vi "DHTxx Temp-Humidity Sensor.vi"   [LabVIEW 2014]
uses:
  QwaveSys_Interface/QwaveSys_Interface.lvlib
  QwaveSys_ESP8266/QwaveSys_ESP8266.lvlib
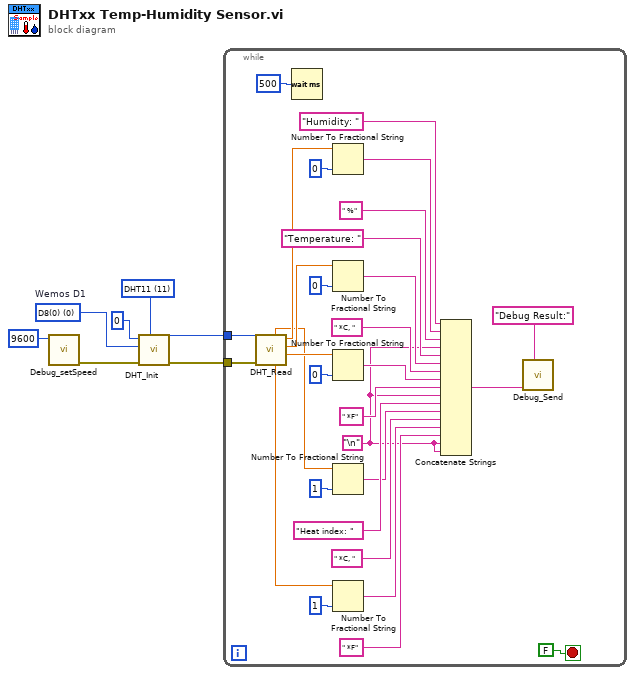
[diagram p0: block diagram]
diagram:
  w2 = u8 0 items=["D0-RX(3)"=3, "D1-TX(1)"=1, "D2(16)"=16, "D3/D15/SCL(5)"=5, "D4/D14/SDA(4)"=4, "D5/D13/SCK(14)-(LED)"=14, "D6/D12/MISO(12)"=12, "D7/D11/MOSI(13)"=13, "D8(0)"=0, "D9/TX1(2)"=2, "D10/SS (15)"=15, "ADC0,(17)"=17]  # Wemos D1
  w4 = u16 11 items=["DHT11"=11, "DHT21"=21, "DHT22"=22] ("Type")
  n1 = call "Debug_setSpeed.vi"("Speed"=u32 9600) -> ("error out"=w1:errorcluster)  [unwired: 10 in]
  n2 = call "DHT_Init.vi"("Type"=w4, "error in (no error)"=w1, "PIN"=w2, "Interface (0-4)"=u8 0) -> ("error out"=w6:errorcluster, "Instance"=w5:u8)  [unwired: 6 in]
  n3 = while {
    tunnel: w6 -> [w37]
    tunnel: w5 -> [w8]
    stop <- FALSE stop-if-true
    w11 = "\n" ("Line Feed Constant")
    n4 = call "DHT_Read.vi"("Instance"=w8, "error in (no error)"=w37) -> ("Fahrenheit"=w24:dbl, "Celsius"=w25:dbl, "Humidity"=w31:dbl, "Heat Index (Fahrenheit)"=w22:dbl, "Heat Index (Celsius)"=w23:dbl)  [unwired: 4 in, 1 out]
    n5 = Wait (ms)(milliseconds to wait=u32 500) -> ()  [unwired: 1 out]
    n6 = Number To Fractional String(number=w31, precision (6)=i16 0) -> (F-format string=w30:string)  [unwired: 2 in]
    n7 = Number To Fractional String(number=w25, precision (6)=i16 0) -> (F-format string=w20:string)  [unwired: 2 in]
    n8 = Number To Fractional String(number=w24, precision (6)=i16 0) -> (F-format string=w18:string)  [unwired: 2 in]
    n9 = Number To Fractional String(number=w23, precision (6)=i16 1) -> (F-format string=w15:string)  [unwired: 2 in]
    n10 = Number To Fractional String(number=w22, precision (6)=i16 1) -> (F-format string=w13:string)  [unwired: 2 in]
    n11 = Concatenate Strings("Humidity: " ("string"), w30, " %" ("string"), w11, "Temperature: " ("string"), w20, " *C, " ("string"), w18, " *F" ("string"), w11, "Heat index: " ("string"), w15, " *C, " ("string"), w13, " *F" ("string"), w11, w11) -> (w10:string)
    n12 = call "Debug_Send.vi"("Name"="Debug Result:", "DATA"=w10) -> ()  [unwired: 10 in]
  }
